vi "AndorIdle.vi"(8 "error in (no error)":errorcluster) -> (0 "error out":errorcluster, 3 "Boolean":bool)   [LabVIEW 2018, in "AndorOWN.lvlib"]
uses:
  AndorOWN.lvlib
  Andor SDK/AndorSDK.lvlib
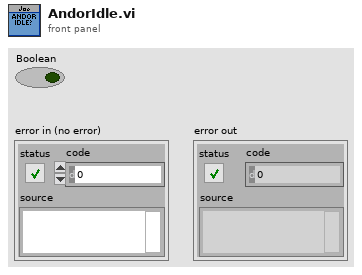
[diagram p1: front panel]
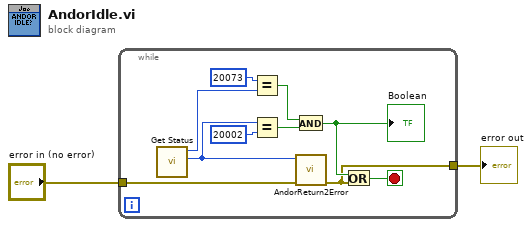
[diagram p0: block diagram]
diagram:
  n1 = while {
    tunnel: "error in (no error)" -> [w5]
    tunnel: [w3] -> w1
    stop <- w4 stop-if-true
    n2 = call "Get Status.vi"() -> ("function return"=w6:u32, "status out"=w10:i32)  [unwired: 10 in]
    n3 = Equal?(x=20073 ("status out"), y=w10) -> (x = y?=w11:bool)
    n4 = Equal?(x=w6, y=20002 ("x")) -> (x = y?=w12:bool)
    n5 = And(x=w11, y=w12) -> (x .and. y?=w7:bool)
    "Boolean" <- w7
    n6 = call "AndorReturn2Error.vi"("error in (no error)"=w5, "Camera return"=w6) -> ("error out"=w3:errorcluster)  [unwired: 9 in]
    n7 = Or(x=w7, y=w3) -> (x .or. y?=w4:bool)
  }
  "error out" <- w1
